vi "Store_File_data.vi"() -> ()   [LabVIEW 2023]
uses:
  Library_Controls/Mode.ctl
  File_Handler_Library.lvlib
panel:
  in  "Save_File_Path":path
  in  "Folder_Info_Path":path
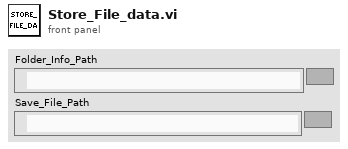
[diagram p1: front panel]
types:
  T1 = typedef "File_Handler_Library.lvlib/Mode.ctl" = enum16{"Write", "Read"}
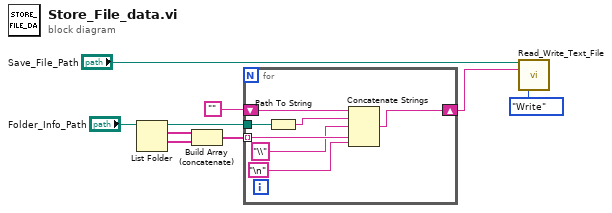
[diagram p0: block diagram]
diagram:
  n1 = List Folder(path="Folder_Info_Path") -> (path out=w8:path, filenames=w7:string[], folder names=w6:string[])  [unwired: 3 in, 1 out]
  n2 = Build Array (concatenate)(w7, w6) -> (w5:string[])
  n3 = for {
    tunnel: w8 -> [w16]
    tunnel: w5 -> [w11] mode=indexing
    shift-right: [w14] -> w1
    shift-left: "" -> [w13]
    n4 = Path To String(path=w16) -> (string=w15:string)
    n5 = Concatenate Strings(w13, w15, "\\", w11, "\n") -> (w14:string)
  }
  n6 = call "Read_Write_Text_File.vi"("File_Path_In"="Save_File_Path", "Data_In"=w1, "Mode"=Mode."Write") -> ()  [unwired: 10 in, 3 out]
